vi "GetWindowSize.vi"(8 "No Error":errorcluster, 11 "Window [SDL_Window *]":i64 format="%.0x") -> (0 "Error Out":errorcluster, 2 "h":i32, 3 "w":i32)   [LabVIEW 2024, in "SDL3.lvlib" / "Video.lvlib"]
doc: "<B>Summary</B>\nGet the size of a window's client area.\n\n<B>Remarks</B>\nThe window pixel size may differ from its window coordinate size if the window is on a high pixel density display. Use <B>SDL_GetWindowSizeInPixels()</B> or <B>SDL_GetRenderOutputSize()</B> to get the real client area size in pixels."
uses:
  Video.lvlib
  Lib/SDL3.dll
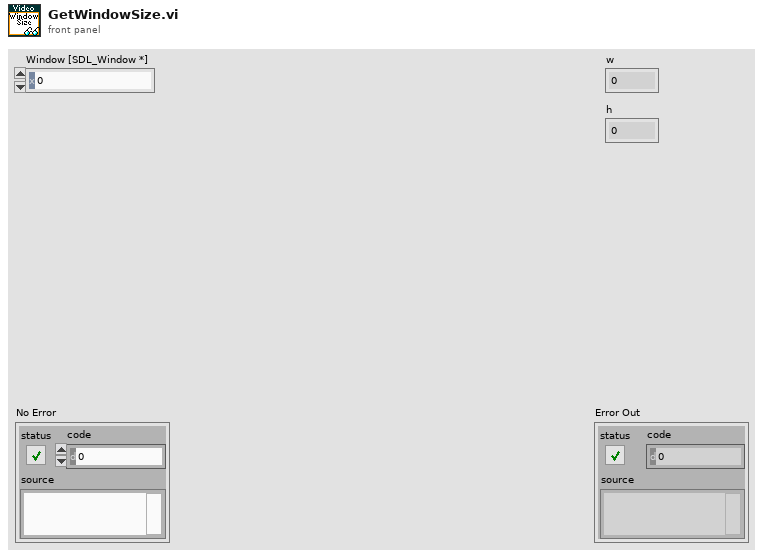
[diagram p1: front panel]
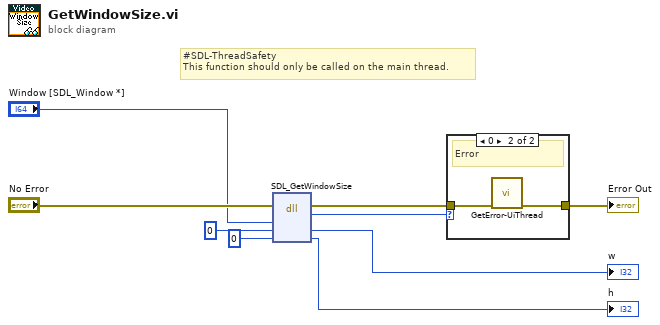
[diagram p0: block diagram]
diagram:
  # "#SDL-ThreadSafety\nThis function should only be called on the main thread."
  n1 = dll-call lib="C:/Users/Thomas/Documents/Projects/LV-SDL3/Sources/SDL3/Lib/SDL3.*" fn="SDL_GetWindowSize"(error in="No Error", "window"="Window [SDL_Window *]", "w"=0 ("W"), "h"=0 ("H")) -> (error out=w4:errorcluster, "return type"=w3:i32, "w"=→"w":i32, "h"=→"h":i32)  [unwired: 3 in, 1 out]
  n2 = case shown="0" w3 {
    tunnel: w4 -> [w10 w12]
    tunnel: [w10 w11] -> w8
    frame Default {
      # "Ok"
    }
    frame 0 {
      # "Error"
      n3 = call "GetError-UiThread.vi"("No Error"=w12) -> ("error out"=w11:errorcluster)  [unwired: 10 in]
    }
  }
  "Error Out" <- w8
